vi "Add Single.vi"(0 "UI in":refnum<class "Assembly Run.lvclass">, 1 "Settings":T4, 5 "Routine":T2=enum."Release Syringe", 7 "Assembly Type":string, 9 "Fixture":T3, 11 "error in (no error)":errorcluster, 12 "Input Settings":T1, 13 "Auto":bool) -> (4 "UI out":refnum<class "Assembly Run.lvclass">, 15 "error out":errorcluster)   [LabVIEW 2021, in "Assembly Run.lvclass"]
uses:
  Assembly Run.lvclass
  Routine/Settings.ctl
  Workspace/Fixture Enum.ctl
  Routine/Routine Enum.ctl
  Routine/Routine.lvclass
  Workspace/Fixture.lvclass
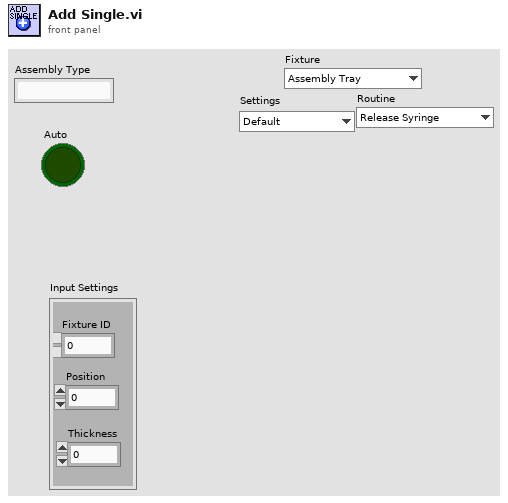
[diagram p1: front panel]
types:
  T1 = cluster{"Fixture ID":dbl, "Position":dbl, "Thickness":dbl}
  T2 = typedef "Routine.lvclass/Routine Enum.ctl" = enum16{"Primary Pick Up", "Secondary Pick Up", "Put Down All", "Secure Syringe", "Release Syringe", "Dispense Epoxy", "Pick Up All", "Put Down Secondary", "Full Assembly"}
  T3 = typedef "Fixture.lvclass/Fixture Enum.ctl" = enum16{"Assembly Tray", "Syringe Space", "Component", "Pick Up Tool", "Current Position"}
  T4 = typedef "Routine.lvclass/Settings.ctl" = enum16{"Default", "Custom"}
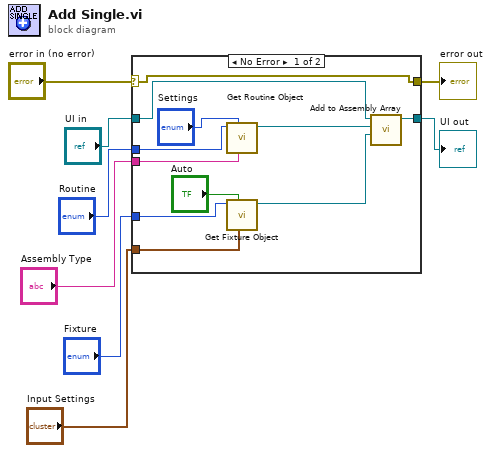
[diagram p0: block diagram]
diagram:
  n1 = case shown="No Error" "error in (no error)" {
    selector: "error in (no error)" -> [w19 w21]
    tunnel: [w19 w21] -> w7
    tunnel: "UI in" -> [w18 w20]
    tunnel: [w17 w20] -> w5
    tunnel: "Fixture" -> [w14 _]
    tunnel: "Routine" -> [w12 _]
    tunnel: "Assembly Type" -> [w11 _]
    tunnel: "Input Settings" -> [w9 _]
    frame No Error {
      n2 = call "Get Routine Object.vi"("Assembly Type"=w11, "Settings"="Settings", "Routine"=w12) -> ("Routine out"=w16:refnum<class "Routine.lvclass">)  [unwired: 7 in, 1 out]
      n3 = call "Get Fixture Object.vi"("Input Settings"=w9, "Auto"="Auto", "Fixture"=w14) -> ("Workspace.lvclass"=w13:refnum<class "Fixture.lvclass">)  [unwired: 6 in, 2 out]
      n4 = call "Add to Assembly Array.vi"("Workspace In"=w13, "Routine In"=w16, "Assembly Run in"=w18) -> ("Assembly Run out"=w17:refnum<class "Assembly Run.lvclass">)  [unwired: 7 in, 1 out]
    }
    frame Error {
    }
  }
  "error out" <- w7
  "UI out" <- w5
